vi "Timer with Error Handling.vi"(6 "Reset":bool, 8 "error in (no error)":errorcluster, 11 "Timeout (ms)":u32) -> (0 "error out":errorcluster, 2 "Elapsed Time (ms)":u32, 3 "Timer Elapsed?":bool)   [LabVIEW 2010]
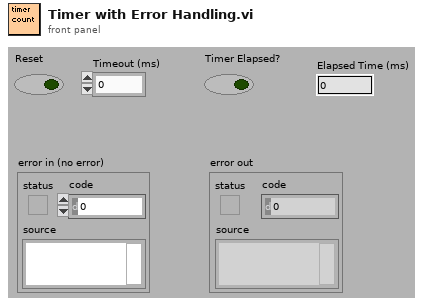
[diagram p1: front panel]
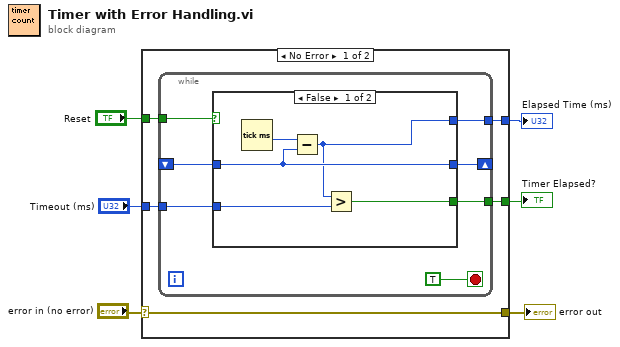
[diagram p0: block diagram]
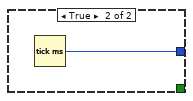
[diagram p2: hidden frame]
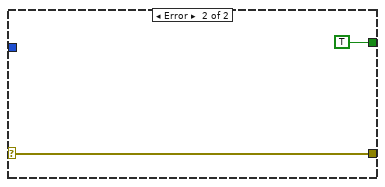
[diagram p3: hidden frame]
diagram:
  n1 = case shown="No Error" "error in (no error)" {
    selector: "error in (no error)" -> [w11 w26]
    tunnel: [w11 w26] -> w5
    tunnel: "Reset" -> [w10 _]
    tunnel: "Timeout (ms)" -> [w9 _]
    tunnel: [w8 TRUE] -> w2
    tunnel: [w7 _] -> w1
    frame No Error {
      n2 = while {
        shift-right: [w17] -> _
        shift-left: _ -> [w15]
        tunnel: w10 -> [w16]
        tunnel: w9 -> [w14]
        tunnel: [w13] -> w8
        tunnel: [w12] -> w7
        stop <- TRUE stop-if-true
        n3 = case shown="False" w16 {
          tunnel: [w22 w24] -> w17
          tunnel: w15 -> [w22 _]
          tunnel: w14 -> [w21 _]
          tunnel: [w20 _] -> w13
          tunnel: [w19 _] -> w12
          frame False {
            n4 = Tick Count (ms)() -> (millisecond timer value=w23:u32)
            n5 = Subtract(x=w23, y=w22) -> (x-y=w19:u32)
            n6 = Greater?(x=w19, y=w21) -> (0:w20:bool)
          }
          frame True {
            n7 = Tick Count (ms)() -> (millisecond timer value=w24:u32)
          }
        }
      }
    }
    frame Error {
    }
  }
  "error out" <- w5
  "Timer Elapsed?" <- w2
  "Elapsed Time (ms)" <- w1
